vi "MCL Device Attached.vi"(10 "handle":i32, 11 "milliseconds":i32) -> (3 "function return":bool)   [LabVIEW 2017, in "Madlib.lvlib"]
doc: "MADLIB_API bool MCL_DeviceAttached(int milliseconds, int handle);"
uses:
  Madlib.lvlib
  Madlib.dll
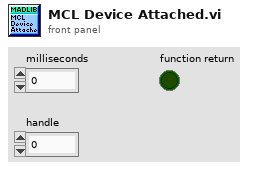
[diagram p1: front panel]
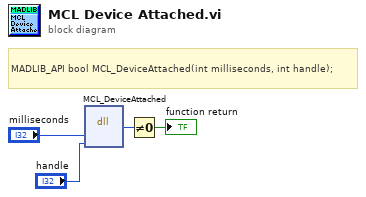
[diagram p0: block diagram]
diagram:
  # "MADLIB_API\tbool\tMCL_DeviceAttached(int milliseconds, int handle);"
  n1 = dll-call lib="C:/Users/francesco/dev/pump-probe/Piezo/lvlib/Madlib.*" fn="MCL_DeviceAttached"("milliseconds"="milliseconds", "handle"="handle") -> (w3:u8)  [unwired: 5 in, 2 out]
  n2 = Not Equal To 0?(x=w3) -> (x != 0?=→"function return":bool)
